vi "which_day.vi"(0 "Hour":u64) -> (1 "which array":i32, 2 "New Date":T1)   [LabVIEW 2011]
uses:
  <vilib>/Utility/miscctls.llb/LVDateTimeRec.ctl
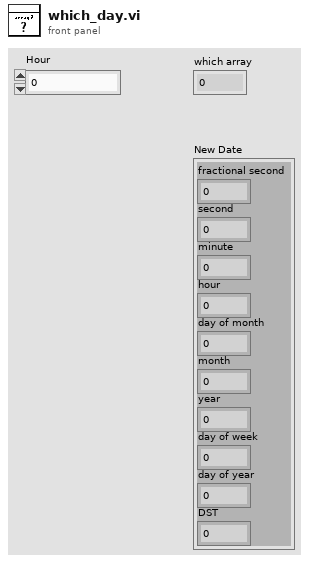
[diagram p1: front panel]
types:
  T1 = typedef "LVDateTimeRec.ctl" = cluster{"fractional second":dbl, "second":i32, "minute":i32, "hour":i32, "day of month":i32, "month":i32, "year":i32, "day of week":i32, "day of year":i32, "DST":i32}
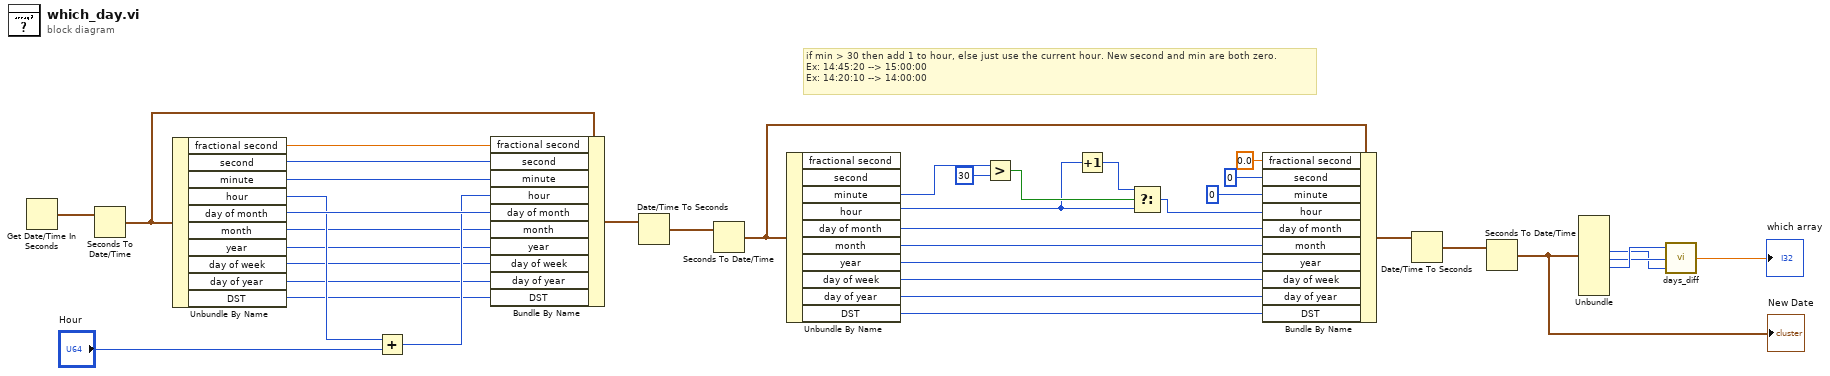
[diagram p0: block diagram]
diagram:
  # "if min > 30 then add 1 to hour, else just use the current hour. New second and min are both zero.\nEx: 14:45:20 --> 15:00:00\nEx: 14:20:10 --> 14:00:00"
  n1 = Get Date/Time In Seconds() -> (seconds since 1Jan1904=w35:timestamp)
  n2 = Seconds To Date/Time(time stamp (now)=w35) -> (date time rec=w38:T1)  [unwired: 1 in]
  n3 = Unbundle By Name(w38) -> ("fractional second"=w26:dbl, "second"=w27:i32, "minute"=w28:i32, "hour"=w37:i32, "day of month"=w39:i32, "month"=w29:i32, "year"=w30:i32, "day of week"=w31:i32, "day of year"=w32:i32, "DST"=w33:i32)
  n4 = Add(x=w37, y="Hour") -> (x+y=w36:u64)
  n5 = Bundle By Name(cluster=w38, "fractional second"=w26, "second"=w27, "minute"=w28, "hour"=w36, "day of month"=w39, "month"=w29, "year"=w30, "day of week"=w31, "day of year"=w32, "DST"=w33) -> (w34:T1)
  n6 = Date/Time To Seconds(2:w34) -> (0:w25:timestamp)  [unwired: 1 in]
  n7 = Seconds To Date/Time(time stamp (now)=w25) -> (date time rec=w2:T1)  [unwired: 1 in]
  n8 = Unbundle By Name(w2) -> ("minute"=w19:i32, "hour"=w12:i32, "day of month"=w11:i32, "month"=w10:i32, "year"=w9:i32, "day of week"=w8:i32, "day of year"=w7:i32, "DST"=w6:i32)  [unwired: 2 out]
  n9 = Greater?(x=w19, y=30) -> (0:w17:bool)
  n10 = Increment(x=w12) -> (x+1=w13:i32)
  n11 = Select(t=w13, s=w17, f=w12) -> (s? t:f=w14:i32)
  n12 = Bundle By Name(cluster=w2, "fractional second"=0.0, "second"=0, "minute"=0, "hour"=w14, "day of month"=w11, "month"=w10, "year"=w9, "day of week"=w8, "day of year"=w7, "DST"=w6) -> (w4:T1)
  n13 = Date/Time To Seconds(2:w4) -> (0:w5:timestamp)  [unwired: 1 in]
  n14 = Seconds To Date/Time(time stamp (now)=w5) -> (date time rec=w1:T1)  [unwired: 1 in]
  "New Date" <- w1
  n15 = Unbundle(w1) -> ("day of month"=w22:i32, "month"=w23:i32, "year"=w24:i32)  [unwired: 7 out]
  n16 = call "days_diff.vi"("day"=w22, "month"=w23, "year"=w24) -> ("Days Diff"=→"which array":dbl)  [unwired: 2 out]
